vi "Probe Drop.vi"(1 "error in (no error)":errorcluster) -> (0 "error out":errorcluster)   [LabVIEW 2021, in "AlliGator Image Profile Window.lvlib"]
doc: "Use this VI to pause any VI containing an error wire, by simply inserting a conditional error probe and selecting pause if error or error code = 0 (no error).\n\nOnce the error probe is removed (i.e. when the diargram is closed, this VI does not interfere with the function of its host VI.\n\nNote: This VI is non-reentrant on purpose, so that it can be used in VIs that are dynamically called. In that case, simply open this VI's diagram and place a probe as instructed. The calling VI can be closed or open, without the Pause.vi being affected."
uses:
  AlliGator/AlliGator Image Profile Window.lvlib
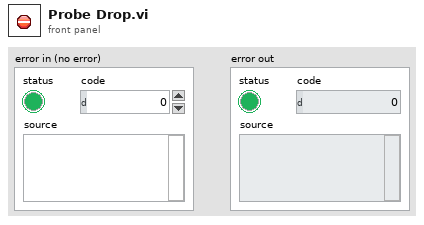
[diagram p1: front panel]
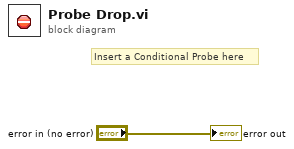
[diagram p0: block diagram]
diagram:
  # "Insert a Conditional Probe here"
  "error out" <- "error in (no error)"
